vi "PH_Stepmotor_BaseClass.Evt Call Reset.vi"(0 "i ref in":refnum<vi>, 1 "Address":T1={"Instance"="N/A", "Motor Nr"=0}, 5 "error in":errorcluster) -> (14 "i ref out":refnum<vi>, 19 "error out":errorcluster)   [LabVIEW 2014, in "PH_Stepmotor_BaseClass.lvlib"]
uses:
  PH_Stepmotor_BaseClass.Axis Address.ctl
  CSCore/CSSystem/CoreLib/CoreLib.int 2 byte array.vi
  PH_Stepmotor_BaseClass.lvlib
  CSCore/BaseProcess/BaseProcess.lvlib
  CSCore/CSSystem/CoreLib/CoreLib.lvlib
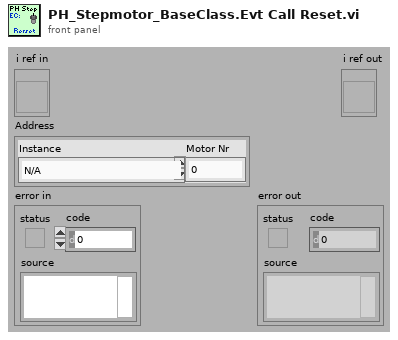
[diagram p1: front panel]
types:
  T1 = typedef "PH_Stepmotor_BaseClass.lvlib/PH_Stepmotor_BaseClass.Axis Address.ctl" = cluster{"Instance":string, "Motor Nr":i32}
  T2 = typedef "CoreDefs.rawDataType.ctl" = i8[]
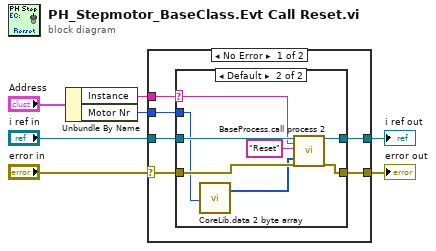
[diagram p0: block diagram]
diagram:
  n1 = Unbundle By Name("Address") -> ("Instance"=w2:string, "Motor Nr"=w1:i32)
  n2 = case shown="No Error" "error in" {
    selector: "error in" -> [w10 w24]
    tunnel: [w13 w24] -> w4
    tunnel: w2 -> [w9 _]
    tunnel: "i ref in" -> [w12 w25]
    tunnel: [w11 w25] -> w6
    tunnel: w1 -> [w8 _]
    frame No Error {
      n3 = case shown="Default" w9 {
        selector: w9 -> [_ w18]
        tunnel: [w15 w23] -> w13
        tunnel: w10 -> [w15 w21]
        tunnel: w12 -> [w14 w20]
        tunnel: [w14 w19] -> w11
        tunnel: w8 -> [_ w17]
        frame "N/A" {
        }
        frame Default {
          n4 = call-poly "CoreLib.data 2 byte array.vi"("i32"=w17) -> ("byteArray out"=w16:T2)  [unwired: 18 in]
          n5 = call "BaseProcess.call process 2.vi"("i ref in"=w20, "Object"=w18, "Selector"="Reset", "Data"=w16, "error in (no error)"=w21) -> ("i ref out"=w19:refnum<vi>, "error out"=w23:errorcluster)  [unwired: 13 in]
        }
      }
    }
    frame Error {
    }
  }
  "i ref out" <- w6
  "error out" <- w4
